vi "Release Control Cluster.vi"(11 "output cluster":T1) -> ()   [LabVIEW 2016, in "Controller.lvclass"]
uses:
  Controller.lvclass
  Controllers.ctl
  Motion/Motion Folder/Motion.lvclass
  I-O/I-O Folder/I-O.lvclass
  Dispenser/Dispenser Folder/Dispenser.lvclass
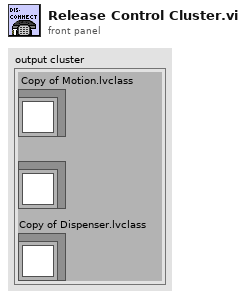
[diagram p1: front panel]
types:
  T1 = typedef "Controller.lvclass/Controllers.ctl" = cluster{"Copy of Motion.lvclass":refnum<class "Motion.lvclass">, "Copy of I-O.lvclass ":refnum<class "I-O.lvclass">, "Copy of Dispenser.lvclass":refnum<class "Dispenser.lvclass">}
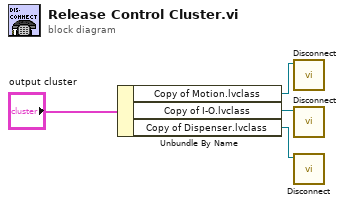
[diagram p0: block diagram]
diagram:
  n1 = Unbundle By Name("output cluster") -> ("Copy of Motion.lvclass"=w3:refnum<class "Motion.lvclass">, "Copy of I-O.lvclass"=w2:refnum<class "I-O.lvclass">, "Copy of Dispenser.lvclass"=w1:refnum<class "Dispenser.lvclass">)
  n2 = call-dynamic "Disconnect.vi"("Motion in"=w3) -> ()  [unwired: 9 in, 1 out]
  n3 = call-dynamic "Disconnect.vi"("I-O in"=w2) -> ()  [unwired: 9 in, 1 out]
  n4 = call-dynamic "Disconnect.vi"("Controller in"=w1) -> ()  [unwired: 9 in, 1 out]
